vi "soundSingleton.vi"(7 "Option":enum16{"Create", "Destroy"}(ring), 8 "error in (no error)":errorcluster, 10 "Sound Parameters":T1={"Device ID"=0, "Volume"=50.0, "frequency"=10.0, "duration (s)"=0.0} {"frequency" format="%0.2p"; "Volume" scale=0.0..100.0}, 11 "Sound in":refnum<class "Sound.lvclass">) -> (0 "error out":errorcluster, 3 "Sound out":refnum<class "Sound.lvclass">)   [LabVIEW 2019, in "Sound.lvclass"]
uses:
  Sound.lvclass
  Sound.lvclass/Sound.ctl
  <vilib>/measure/NI_MABase.lvlib
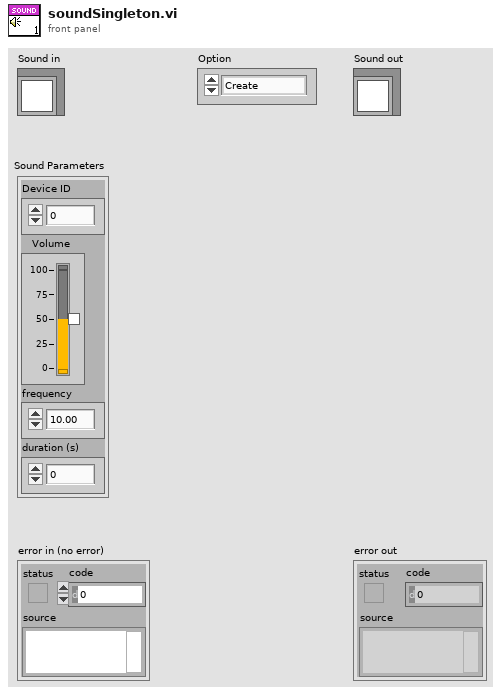
[diagram p1: front panel]
types:
  T1 = cluster{"Device ID":u32, "Volume":dbl, "frequency":dbl, "duration (s)":dbl}
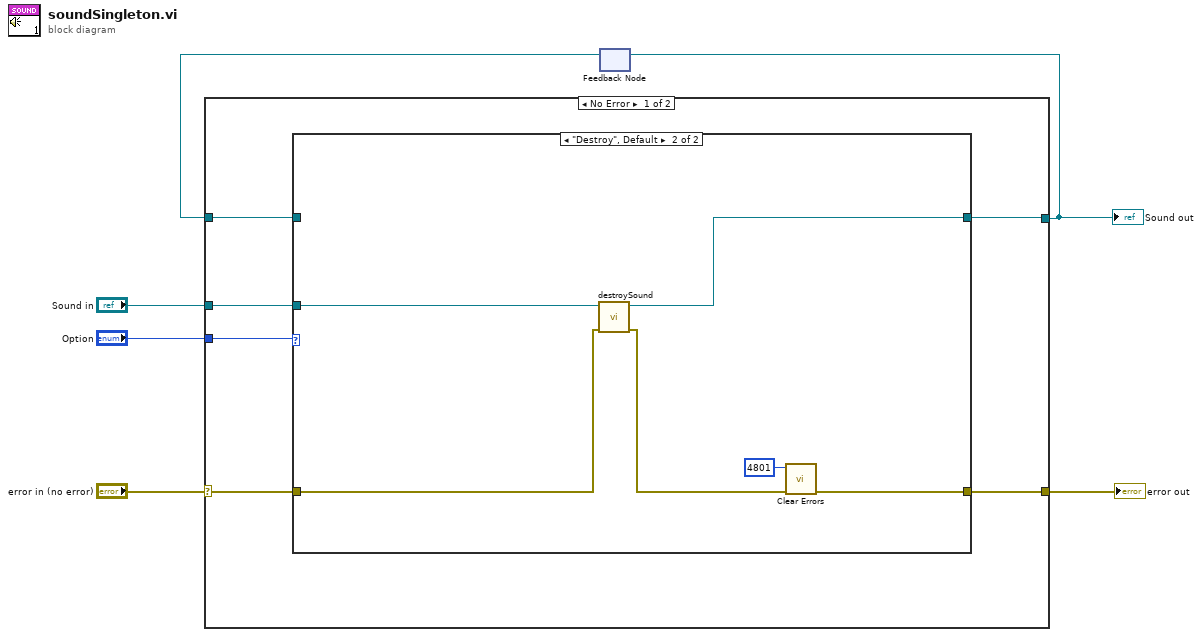
[diagram p0: block diagram]
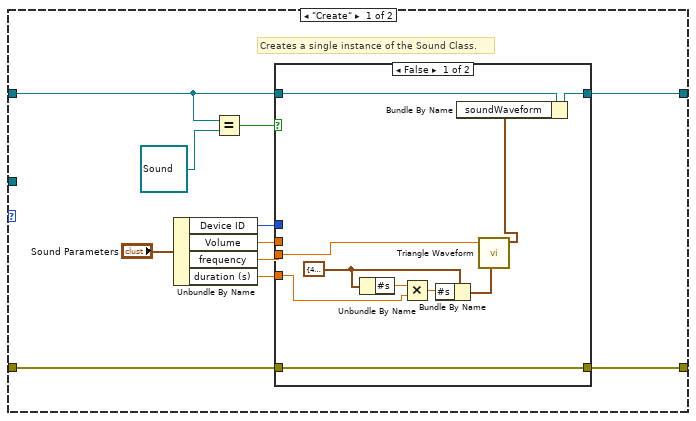
[diagram p2: hidden frame]
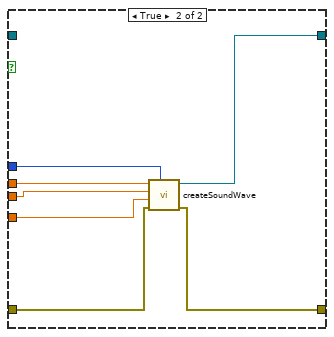
[diagram p3: hidden frame]
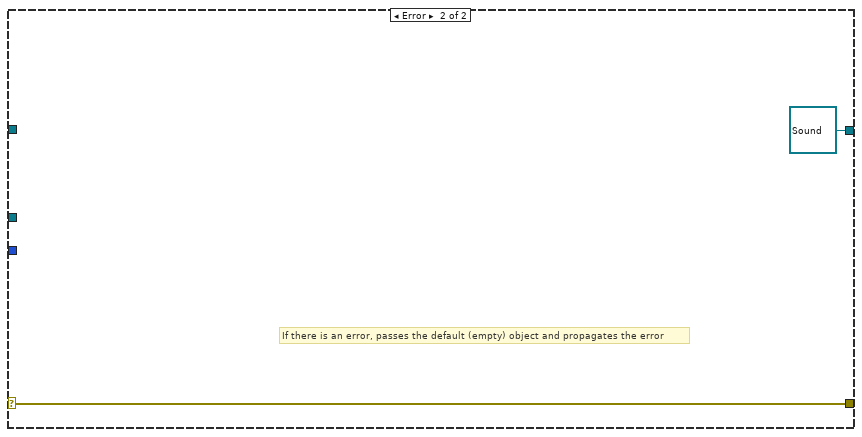
[diagram p4: hidden frame]
diagram:
  n1 = feedback #1() -> (w2:refnum<class "Sound.lvclass">)  [unwired: 1 in]
  n2 = case shown="No Error" "error in (no error)" {
    selector: "error in (no error)" -> [w9 w48]
    tunnel: [w10 w48] -> w5
    tunnel: w2 -> [w12 _]
    tunnel: [w11 refnum<class "Sound.lvclass"> refnum ("Sound out")] -> w4
    tunnel: "Option" -> [w8 _]
    tunnel: "Sound in" -> [w7 _]
    frame No Error {
      n3 = case shown="\"Destroy\", Default" w8 {
        tunnel: w12 -> [w22 _]
        tunnel: [w21 w43] -> w11
        tunnel: [w20 w42] -> w10
        tunnel: w9 -> [w19 w46]
        tunnel: w7 -> [_ w44]
        frame "Create" {
          # "Creates a single instance of the Sound Class."
          n4 = Unbundle By Name("Sound Parameters") -> ("Device ID"=w16:u32, "Volume"=w15:dbl, "frequency"=w14:dbl, "duration (s)"=w13:dbl)
          n5 = Equal?(x=w22, y=refnum<class "Sound.lvclass"> refnum ("Sound.lvclass")) -> (x = y?=w23:bool)
          n6 = case shown="False" w23 {
            tunnel: w22 -> [w33 _]
            tunnel: [w25 w40] -> w21
            tunnel: [w32 w39] -> w20
            tunnel: w19 -> [w32 w38]
            tunnel: w16 -> [_ w37]
            tunnel: w15 -> [_ w36]
            tunnel: w14 -> [w26 w35]
            tunnel: w13 -> [w27 w34]
            frame False {
              w30 = cluster{"Fs":dbl, "#s":dbl} {"Fs"=44100.0, "#s"=44100.0} ("sampling info")
              n7 = Unbundle By Name(w30) -> ("#s"=w31:dbl)
              n8 = Multiply(x=w31, y=w27) -> (x*y=w29:dbl)
              n9 = Bundle By Name(cluster=w30, "#s"=w29) -> (w28:cluster{"Fs":dbl, "#s":dbl})
              n10 = call <vilib>:"Triangle Waveform.vi"("sampling info"=w28, "frequency"=w26) -> ("signal out"=w24:waveform(dbl))  [unwired: 8 in, 1 out]
              n11 = Bundle By Name(cluster=w33, "soundWaveform"=w24) -> (w25:refnum<class "Sound.lvclass">)
            }
            frame True {
              n12 = call "createSoundWave.vi"("Device ID"=w37, "error in (no error)"=w38, "duration (s)"=w34, "frequency"=w35, "Volume"=w36) -> ("error out"=w39:errorcluster, "Sound out"=w40:refnum<class "Sound.lvclass">)  [unwired: 5 in]
            }
          }
        }
        frame "Destroy", Default {
          n13 = call "destroySound.vi"("error in (no error)"=w46, "Sound in"=w44) -> ("error out"=w45:errorcluster, "Sound out"=w43:refnum<class "Sound.lvclass">)  [unwired: 8 in]
          n14 = call <vilib>:"Clear Errors.vi"("error in (no error)"=w45, "specific error code to clear (0: all)"=4801) -> ("error out"=w42:errorcluster)  [unwired: 4 in, 1 out]
        }
      }
    }
    frame Error {
      # "If there is an error, passes the default (empty) object and propagates the error"
    }
  }
  "error out" <- w5
  "Sound out" <- w4
  n15 = feedback-in #1(w4) -> ()
